vi "send_peakcenter_to_AnalysisObj.vi"(0 "SessionID":string, 5 "isotope name":string, 7 "peak center value":string, 11 "error in (no error)":errorcluster) -> (15 "error out":errorcluster)   [LabVIEW 2018]
doc: "sends the peak center data to the AnalysisSession (SessionID) and stores them in the peak center array"
uses:
  Classes/Analysis/Analysis.lvclass
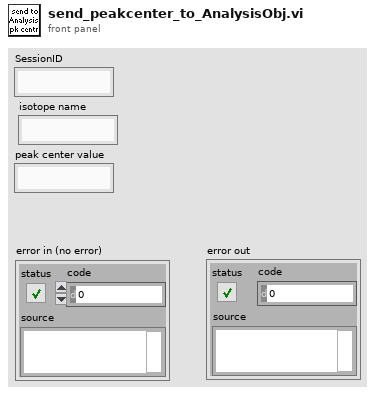
[diagram p1: front panel]
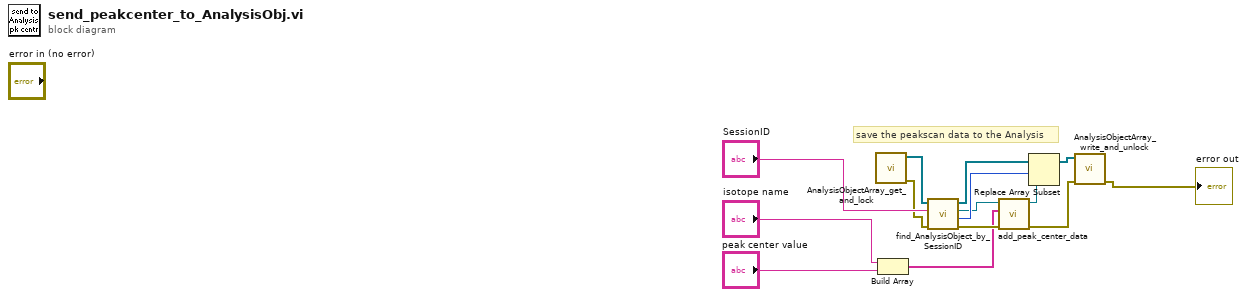
[diagram p0: block diagram]
diagram:
  # "save the peakscan data to the Analysis"
  n1 = call "AnalysisObjectArray_get_and_lock.vi"() -> ("error out"=w7:errorcluster, "AnalysisObjects"=w4:refnum<class "Analysis.lvclass">[])  [unwired: 10 in]
  n2 = Build Array("isotope name", "peak center value") -> (w3:string[])
  n3 = call "find_AnalysisObject_by_SessionID.vi"("error in (no error)"=w7, "SessionID"="SessionID", "AnalysisObjects in"=w4) -> ("error out"=w6:errorcluster, "index of found"=w10:i32, "found AnalyisObject"=w5:refnum<class "Analysis.lvclass">, "AnalysisObjects out"=w8:refnum<class "Analysis.lvclass">[])  [unwired: 5 in]
  n4 = call-dynamic "add_peak_center_data.vi"("error in (no error)"=w6, "peakcenter data"=w3, "Analysis in"=w5) -> ("error out"=w12:errorcluster, "Analysis out"=w9:refnum<class "Analysis.lvclass">)  [unwired: 7 in]
  n5 = Replace Array Subset(array=w8, new element=w9, index=w10) -> (w11:refnum<class "Analysis.lvclass">[])
  n6 = call "AnalysisObjectArray_write_and_unlock.vi"("error in (no error)"=w12, "AnalysisObjects"=w11) -> ("error out"=→"error out":errorcluster)  [unwired: 9 in]
